vi "Stop Core.vi"(10 "final error code":i32, 11 "Appearance Actor in":refnum<class "Appearance Actor.lvclass">) -> (3 "Appearance Actor out":refnum<class "Appearance Actor.lvclass">)   [LabVIEW 2021, in "Appearance Actor.lvlib" / "Appearance Actor.lvclass"]
doc: "In addition to the following, this method also sends a message to the monitor to notify it that the actor has stopped execution.\n\n(<B>Filename</B>: Actor Framework.lvlib:Actor.lvclass:Stop Core.vi)\n\nDefines what the actor does before it stops. Use the <B>final error code</B> input to determine whether the actor shut down in response to an error.\n\nBy default, this method does nothing. A descendant class may override it to define behavior, such as shutting down any processes the actor initiated in its override of the Actor Core method.\n\nCopyright: MGI\n\nAuthored by Derek Trepanier\nsupport@mooregoodideas.com\nwww.mooregoodideas.com\n\nCopyright (c) 2014, Moore Good Ideas, Inc.\n\nAll rights reserved.\n\nRedistribution and use in source and binary forms, with or without modification, are permitted provided that the following conditions are met:\n\n * Redistributions of source code must retain the above copyright notice, this list of conditions and the following disclaimer.\n * Redistributions in binary form must reproduce the above copyright notice, this list of conditions and the following disclaimer in the documentation and/or other materials provided with the distribution.\n * Neither the name of Moore Good Ideas, Inc. nor the names of its contributors may be used to endorse or promote products derived from this software without specific prior written permission.\n\nTHIS SOFTWARE IS PROVIDED BY THE COPYRIGHT HOLDERS AND CONTRIBUTORS \"AS IS\" AND ANY EXPRESS OR IMPLIED WARRANTIES, INCLUDING, BUT NOT LIMITED TO, THE IMPLIED WARRANTIES OF MERCHANTABILITY AND FITNESS FOR A PARTICULAR PURPOSE ARE DISCLAIMED. IN NO EVENT SHALL THE COPYRIGHT OWNER OR CONTRIBUTORS BE LIABLE FOR ANY DIRECT, INDIRECT, INCIDENTAL, SPECIAL, EXEMPLARY, OR CONSEQUENTIAL DAMAGES (INCLUDING, BUT NOT LIMITED TO, PROCUREMENT OF SUBSTITUTE GOODS OR SERVICES; LOSS OF USE, DATA, OR PROFITS; OR BUSINESS INTERRUPTION) HOWEVER CAUSED AND ON ANY THEORY OF LIABILITY, WHETHER IN CONTRACT, STRICT LIABILITY, OR TORT (INCLUDING NEGLIGENCE OR OTHERWISE) ARISING IN ANY WAY OUT OF THE USE OF THIS SOFTWARE, EVEN IF ADVISED OF THE POSSIBILITY OF SUCH DAMAGE."
uses:
  Appearance Actor.lvclass
  C:/Program Files (x86)/National Instruments/LabVIEW 2021/vi.lib/ActorFramework/Actor/Actor.lvclass
  <vilib>/ActorFramework/Message Enqueuer/Message Enqueuer.lvclass
  <vilib>/ActorFramework/Actor/Actor.lvclass/Actor.ctl
  Appearance Actor.lvclass/Appearance Actor.ctl
  Theme Classes/Generic Theme/Generic Theme.lvclass
  <vilib>/MGI/Panel Manager/Panel Actor/Panel Actor/Panel Actor.lvclass
  <vilib>/ActorFramework/Actor/Actor.lvclass
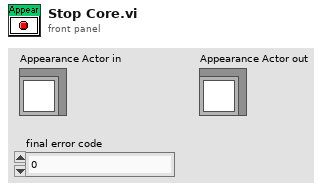
[diagram p1: front panel]
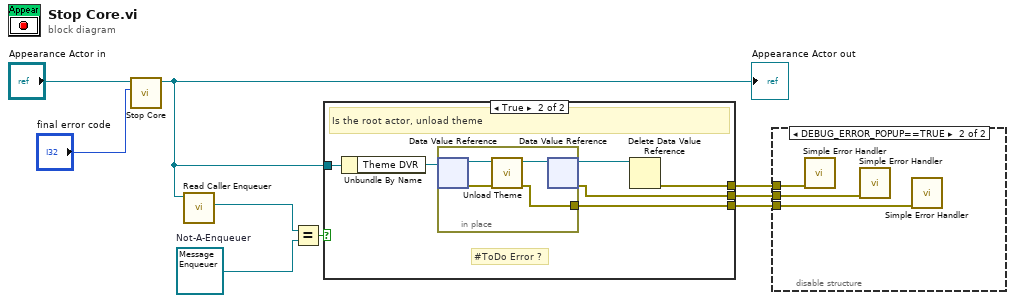
[diagram p0: block diagram]
diagram:
  w6 = refnum<class "Message Enqueuer.lvclass"> refnum  # Not-A-Enqueuer
  n1 = call-parent "Stop Core.vi"("final error code"="final error code", "Monitored Actor in"="Appearance Actor in") -> ("Monitored Actor out"=w5:refnum<class "Appearance Actor.lvclass">)  [unwired: 9 in]
  "Appearance Actor out" <- w5
  n2 = call <vilib>:"Read Caller Enqueuer.vi"("Actor"=w5) -> ("Caller Enqueuer"=w7:refnum<class "Message Enqueuer.lvclass">)  [unwired: 10 in]
  n3 = Equal?(x=w7, y=w6) -> (x = y?=w4:bool)
  n4 = case shown="True" w4 {
    tunnel: w5 -> [_ w15]
    tunnel: [_ w12] -> w3
    tunnel: [_ w11] -> w2
    tunnel: [_ w10] -> w1
    frame False {
    }
    frame True {
      # "#ToDo Error ?"
      # "Is the root actor, unload theme"
      n5 = Unbundle By Name(w15) -> ("Theme DVR"=w14:refnum<data-value>)
      n6 = in-place {
        in-place-border: [w16] -> w10
        n7 = in-place-dvr #1(w14) -> (w19:refnum<class "Generic Theme.lvclass">, w18:errorcluster)
        n8 = call-dynamic "Unload Theme.vi"("Error In"=w18, "Generic Theme in"=w19) -> ("Error Out"=w16:errorcluster, "Generic Theme out"=w17:refnum<class "Generic Theme.lvclass">)  [unwired: 8 in]
        n9 = in-place-dvr #1(w17) -> (w13:refnum<data-value>, w11:errorcluster)
      }
      n10 = Delete Data Value Reference(data value reference=w13) -> (error out=w12:errorcluster)  [unwired: 1 in, 1 out]
    }
  }
  n11 = disable-structure shown="DEBUG_ERROR_POPUP==TRUE" {
    disable-tunnel: w3 -> [_ w22]
    disable-tunnel: w2 -> [_ w21]
    disable-tunnel: w1 -> [_ w20]
    frame condition #0 {
    }
    frame condition #1 (active) {
      n12 = call <vilib>:"Simple Error Handler.vi"("error in (no error)"=w22) -> ()  [unwired: 4 in, 5 out]
      n13 = call <vilib>:"Simple Error Handler.vi"("error in (no error)"=w21) -> ()  [unwired: 4 in, 5 out]
      n14 = call <vilib>:"Simple Error Handler.vi"("error in (no error)"=w20) -> ()  [unwired: 4 in, 5 out]
    }
  }
